vi "Initialize ROV.vi"(8 "error in (no error)":errorcluster, 11 "Device Name":string="Controller (XBOX 360 For Windows)" caption="Give the exact \"divice name\" string of the joypad you would like to use.") -> (0 "error out":errorcluster, 3 "ROV Host.lvclass":refnum<class "ROV Host.lvclass">, 5 "Listed Devices":T1(array[cluster]))   [LabVIEW 2012, in "ROV Host.lvclass"]
uses:
  ROV Host.lvclass
  ROV Host.lvclass/ROV Host.ctl
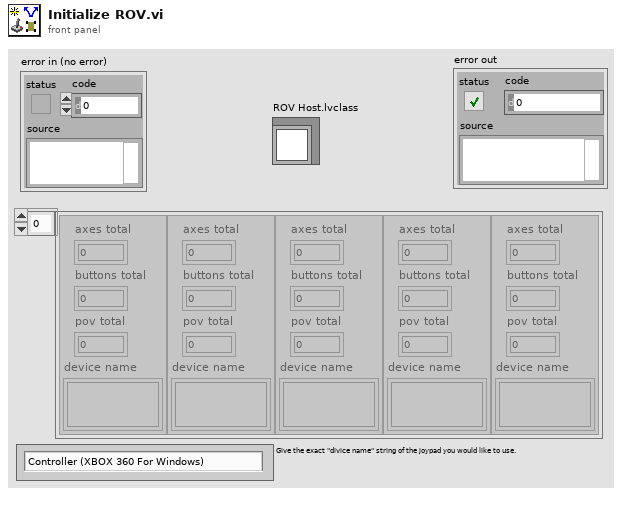
[diagram p1: front panel]
types:
  T1 = cluster{"axes total":u32, "buttons total":u32, "pov total":u32, "device name":string}[]
  T2 = cluster{"device ID":refnum<k1>, "Device Name":string, "axis info":cluster{"X axis":dbl[], "Y axis":dbl[], "Z axis":dbl[], "X axis rotation":dbl[], "Y axis rotation":dbl[], "Z axis rotation":dbl[], "U axis":dbl[], "V axis":dbl[]}}
  T3 = typedef "NI_Robotics_Steering Class Types.lvlib/Mecanum Steering Frame.ctl" = refnum<class "NI_Robotics_Mecanum Steering Frame.lvclass">
  T4 = typedef "NI_Robotics_Steering Class Types.lvlib/Differential Steering Frame.ctl" = refnum<class "NI_Robotics_Differential Steering Frame.lvclass">
  T5 = cluster{"mecanum steering frame out":T3, "differential steering frame out":T4}
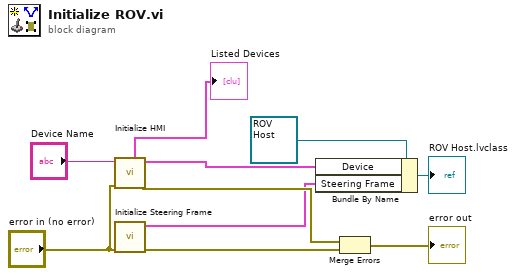
[diagram p0: block diagram]
diagram:
  n1 = call "Initialize HMI.vi"("error in (no error)"="error in (no error)", "Device Name"="Device Name") -> ("error out"=w9:errorcluster, "Device"=w5:T2, "Listed Devices"=→"Listed Devices":T1)  [unwired: 7 in]
  n2 = call "Initialize Steering Frame.vi"("error in (no error)"="error in (no error)") -> ("error out"=w8:errorcluster, "Steering Frame out"=w4:T5)  [unwired: 9 in]
  n3 = Bundle By Name(cluster=refnum<class "ROV Host.lvclass"> refnum ("ROV Host.lvclass"), "Device"=w5, "Steering Frame"=w4) -> (→"ROV Host.lvclass":refnum<class "ROV Host.lvclass">)
  n4 = Merge Errors(w9, w8) -> (→"error out":errorcluster)
